vi "Write Values.vi"(8 "error in (no error)":errorcluster, 10 "Values":dbl[](array[numeric]), 11 "Log Write Message in":refnum<class "Log Write Message.lvclass">) -> (0 "error out":errorcluster, 3 "Log Write Message out":refnum<class "Log Write Message.lvclass">)   [LabVIEW 2020, in "Messaging.lvlib" / "Log Write Message.lvclass"]
uses:
  Log Write Message.lvclass
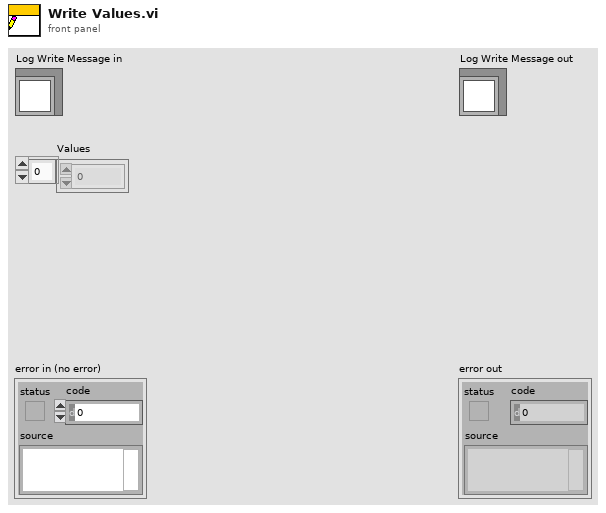
[diagram p1: front panel]
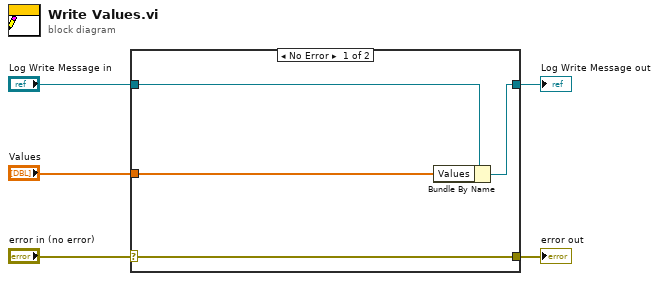
[diagram p0: block diagram]
diagram:
  n1 = case shown="No Error" "error in (no error)" {
    selector: "error in (no error)" -> [w9 w10]
    tunnel: [w9 w10] -> w4
    tunnel: [w7 w11] -> w2
    tunnel: "Log Write Message in" -> [w8 w11]
    tunnel: "Values" -> [w6 _]
    frame No Error {
      n2 = Bundle By Name(cluster=w8, "Values"=w6) -> (w7:refnum<class "Log Write Message.lvclass">)
    }
    frame Error {
    }
  }
  "error out" <- w4
  "Log Write Message out" <- w2
